vi "Format Time.vi"(11 "time (HH:MM:SS)":dbl format="%<%H:%M:%S>t") -> (3 "time string":string)   [LabVIEW 2019, in "Pet Feeder.lvlib"]
uses:
  Pet Feeder.lvlib
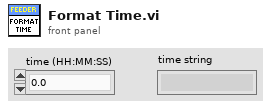
[diagram p1: front panel]
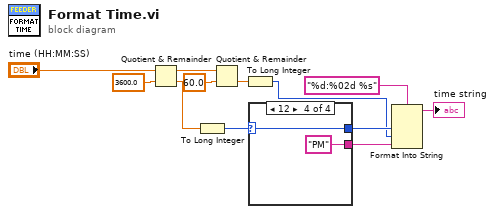
[diagram p0: block diagram]
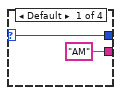
[diagram p2: hidden frame]
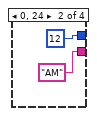
[diagram p3: hidden frame]
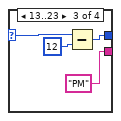
[diagram p4: hidden frame]
diagram:
  n1 = Quotient & Remainder(x="time (HH:MM:SS)", y=3600.0) -> (x-y*floor(x/y)=w10:dbl, floor(x/y)=w8:dbl)
  n2 = To Long Integer(number=w8) -> (32bit integer=w7:i32)
  n3 = Quotient & Remainder(x=w10, y=60.0) -> (floor(x/y)=w6:dbl)  [unwired: 1 out]
  n4 = To Long Integer(number=w6) -> (32bit integer=w3:i32)
  n5 = case shown="12" w7 {
    selector: w7 -> [w13 _ w19 w21]
    tunnel: ["AM" "AM" "PM" "PM"] -> w2
    tunnel: [w13 12 w17 w21] -> w4
    frame Default {
    }
    frame 0, 24 {
    }
    frame 13..23 {
      n6 = Subtract(x=w19, y=12) -> (x-y=w17:i32)
    }
    frame 12 {
    }
  }
  n7 = Format Into String(format string="%d:%02d %s", w4, w3, w2) -> (resulting string=→"time string":string)  [unwired: 2 in, 1 out]
